vi "Update From Selection.vi"(8 "error in":errorcluster, 10 "File Contents":string[](array[string]), 11 "Report Viewer in":refnum<class "Report Viewer.lvclass">) -> (0 "error out":errorcluster, 3 "Report Viewer out":refnum<class "Report Viewer.lvclass">)   [LabVIEW 2023, in "Report Viewer.lvlib" / "Report Viewer.lvclass"]
uses:
  Library/Report Viewer.lvclass
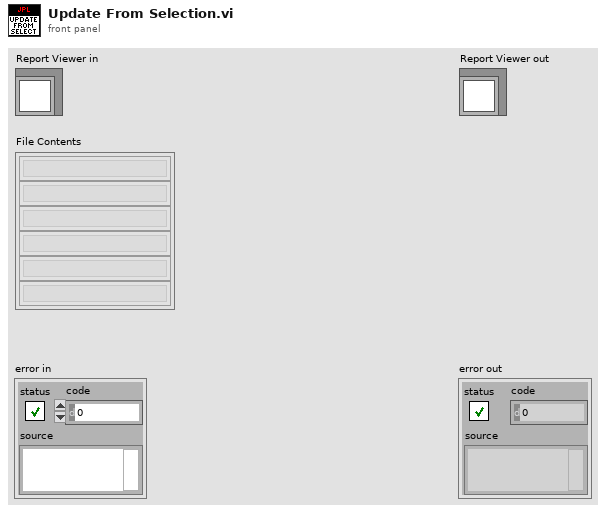
[diagram p1: front panel]
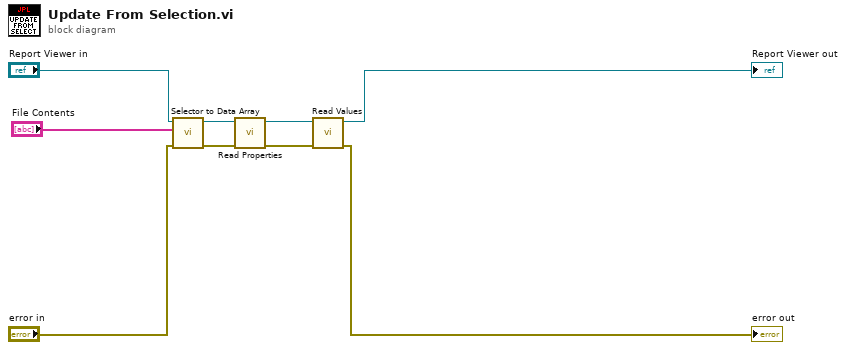
[diagram p0: block diagram]
diagram:
  n1 = call "Selector to Data Array.vi"("error in"="error in", "Selection"="File Contents", "Report Viewer in"="Report Viewer in") -> ("error out"=w9:errorcluster, "Report Viewer out"=w8:refnum<class "Report Viewer.lvclass">)  [unwired: 7 in]
  n2 = call "Read Properties.vi"("error in"=w9, "Report Viewer in"=w8) -> ("error out"=w4:errorcluster, "Report Viewer out"=w3:refnum<class "Report Viewer.lvclass">)  [unwired: 8 in]
  n3 = call "Read Values.vi"("error in"=w4, "Report Viewer in"=w3) -> ("error out"=→"error out":errorcluster, "Report Viewer out"=→"Report Viewer out":refnum<class "Report Viewer.lvclass">)  [unwired: 8 in]
